vi "测试.vi"() -> ()   [LabVIEW 2014, in "XControl.xctl"]
uses:
  XControl.xctl
panel:
  in  "XControl":bool(xcontrol)
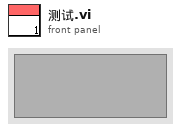
[diagram p1: front panel]
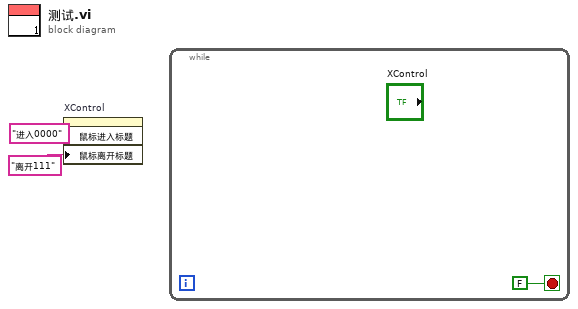
[diagram p0: block diagram]
diagram:
  n1 = property on="XControl" class="XControl (严格)"("鼠标进入标题"="进入0000", "鼠标离开标题"="离开111") -> ()  [unwired: 2 in, 2 out]
  n2 = while {
    stop <- FALSE stop-if-true
  }
